vi "APTpiezoClose.vi"(4 "error in (no error)":errorcluster, 7 "reference":refnum<k7>) -> (0 "error out":errorcluster)   [LabVIEW 2013]
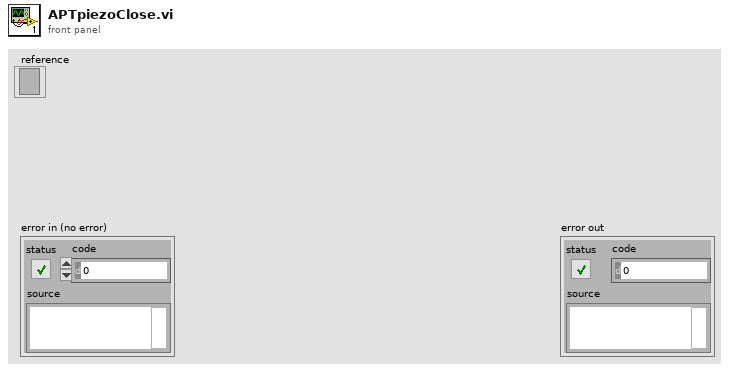
[diagram p1: front panel]
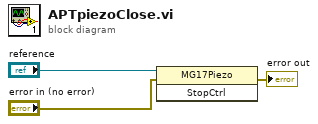
[diagram p0: block diagram]
diagram:
  n1 = invoke class="MG17Piezo" method="StopCtrl"(reference="reference", error in="error in (no error)") -> (error out=→"error out":errorcluster)  [unwired: 1 in, 2 out]
